vi "Functional data-Extract and save.vi"(7 "Simulate":bool, 8 "error in (no error)":errorcluster, 11 "Element received in the queue":T1={"Imaging Protocol"=enum."Live Imaging", "Number of Trials"=0, "Frame Size"=512, "# Averaged frames"=0, "Dwell time (us)"=0.0, "Index of Z-plane"=0, "Timelapse?"=FALSE, "Logging process is active"=FALSE, "Speed logging enabled"=FALSE, "tdms file ref"=refnum, "path"=path "", "Trial Number"=0, "Expected # points acquired"=FALSE, "Manually stopped"=FALSE, "Last trial"=FALSE, "Ch0 data"=[], "Ch1 data"=[], "Ref Data"=[], "Ref Frame Time"=[], "Image Time"=[], "Continuous Time"=[], "Ref X Length"=0, "Ref Y Length"=0, "# Ref Averaged frames"=0, "Ref Dwell time (us)"=0.0, "Points acquired"={"Ch0 last trial"=0, "Ch1 last trial"=0, "All trials"=0}, "HW Timings File"=refnum} {"Ref Dwell time (us)" format="%#.6g"; "Frame Size" items=["100X100"=100, "128X128"=128, "200X200"=200, "256X256"=256, "512X512"=512, "1024x1024"=1024, "2048x2048"=2048]; "Dwell time (us)" format="%#.6g"}) -> (0 "error out":errorcluster, 2 "Destination folder":path)   [LabVIEW 2020]
uses:
  Typedefs/Logging queue element.ctl
  Typedefs/Imaging Protocols enum.ctl
  Typedefs/Frame Size.ctl
  Typedefs/Acquired points count.ctl
  User Interface/Visualisation/Functional Imaging Viewer/SubVIs/Experiment header interface/Typedefs/Header file interface module functions enum.ctl
  User Interface/Visualisation/Functional Imaging Viewer/Typedefs/ROI Save interface cluster.ctl
panel:
  out "size(s) 2":i32[](array[numeric])
  out "ROI Data (header removed)":dbl[][](array[numeric])
  out "Functional imaging TDMS file path & name":path
  out "size(s)":i32[](array[numeric])
  out "No.of Cycles":i32
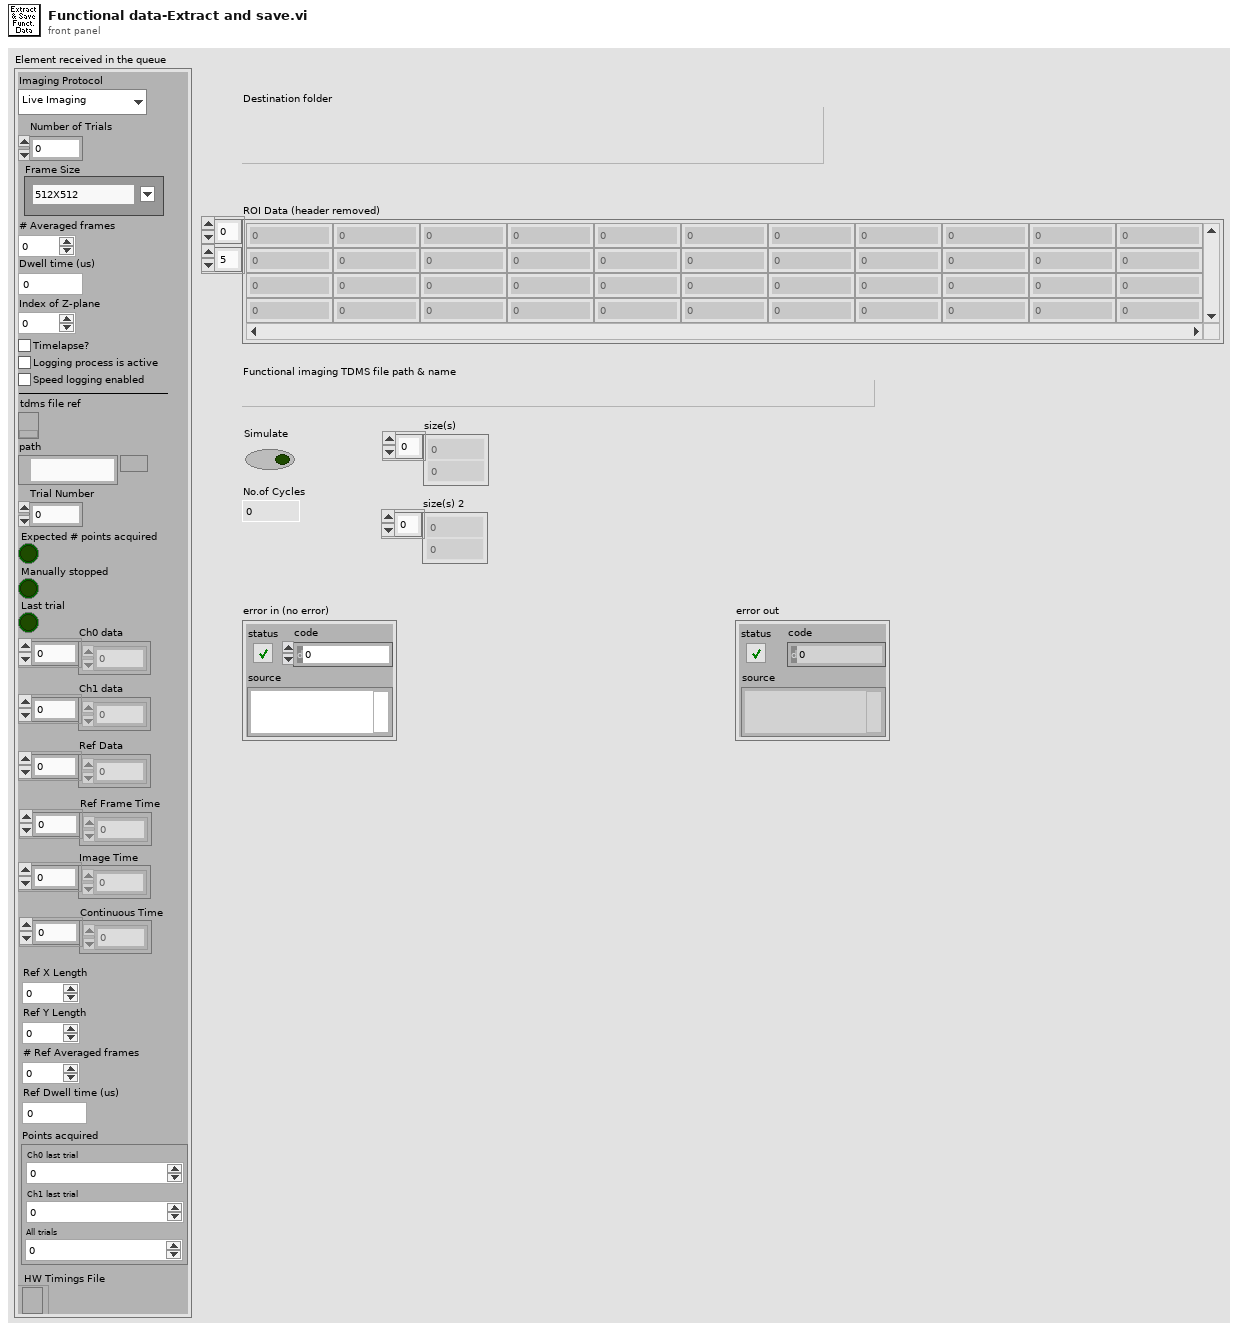
[diagram p1: front panel]
types:
  T1 = typedef "Logging queue element.ctl" = cluster{"Imaging Protocol":T2, "Number of Trials":u16, "Frame Size":T3, "# Averaged frames":u16, "Dwell time (us)":dbl, "Index of Z-plane":i32, "Timelapse?":bool, "Logging process is active":bool, "Speed logging enabled":bool, "tdms file ref":refnum<k34>, "path":path, "Trial Number":i32, "Expected # points acquired":bool, "Manually stopped":bool, "Last trial":bool, "Ch0 data":u32[], "Ch1 data":u32[], "Ref Data":u32[], "Ref Frame Time":u64[], "Image Time":u64[], "Continuous Time":u64[], "Ref X Length":u16, "Ref Y Length":u16, "# Ref Averaged frames":u16, "Ref Dwell time (us)":dbl, "Points acquired":T4, "HW Timings File":refnum<file>}
  T2 = typedef "Imaging Protocols enum.ctl" = enum16{"AOL Z-Stack", "Motor Z Stack", "Functional Acquisition", "Single Plane Acquisition", "Volume Acquisition", "Live Imaging", "Live Plane Imaging", "Live Volume Imaging"}
  T3 = typedef "Frame Size.ctl" = u16
  T4 = typedef "Acquired points count.ctl" = cluster{"Ch0 last trial":u64, "Ch1 last trial":u64, "All trials":u64}
  T5 = typedef "Header file interface module functions enum.ctl" = enum16{"Load experiment header file", "Save experiment header file", "Clear stored values", "Read stored values", "Update specific value in memory", "Update values in memory"}
  T6 = typedef "Header parameters cluster-ALL.ctl" = cluster{"LOGIN":T7, "GLOBAL PARAMETERS":T8, "IMAGING MODES":T10, "TIME SERIES":T11, "MOTOR Z-STACK ":T13, "AOL Z-STACK":T14, "FUNCTIONAL IMAGING":T15, "VOLUME IMAGING":T15, "MOVEMENT CORRECTION":T19, "CALIBRATION":T21, "STATISTICS":T22, "BIOLOGY INFORMATION":T23, "Calibration Data":T24}
  T7 = typedef "Header params -Login.ctl" = cluster{"User":string, "Profile":string, "Software Version":string, "Experiment Date Time":timestamp}
  T8 = typedef "Header params-Global Parameters.ctl" = cluster{"MicroscopeID":string, "Microscope Type":string, "Objective":string, "Field of View (um)":dbl, "Fill time (us)":dbl, "Experiment Type":T9, "Stimuli Trigger":bool, "Speed Logging":bool}
  T9 = typedef "Experiment Type.ctl" = enum16{"In vivo", "In vitro", "Testing", "Calibration", "Other"}
  T10 = typedef "Header params-Imaging Modes.ctl" = cluster{"Time Series":bool, "Motor Zstack":bool, "AOL Zstack":bool, "Functional Imaging":bool, "Volume Imaging":bool}
  T11 = typedef "Header params-Time Series.ctl" = cluster{"Basic Image meta data":T12, "AOL z":dbl}
  T12 = typedef "Header params-Basic image meta data.ctl" = cluster{"Wavelength (nm)":dbl, "# averaged frames":dbl, "laser power (%)":dbl, "Pockels":dbl, "pixel dwell time (us)":dbl, "pmt 1":dbl, "pmt 2":dbl, "back apperture":dbl, "zoom":dbl, "field of view":dbl, "Frame Size":T3, "AOL x centre":dbl, "AOL y centre":dbl, "Stage x position":dbl, "Stage y position":dbl, "Stage z position":dbl}
  T13 = typedef "Header params-Motor Z-stack.ctl" = cluster{"Hdr Basic Image meta data":T12, "Z Start":dbl, "Z Stop":dbl, "No of Planes":i32, "Laser Power (%) at Z Start":dbl, "Laser Power (%) at Z Stop":dbl}
  T14 = typedef "Header params-AOL Z-stack.ctl" = cluster{"Hdr Basic Image meta data":T12, "Z Start":dbl, "Z Stop":dbl, "No of Planes":i32, "Laser Power (%) at Z Start":dbl, "Laser Power (%) at Z Stop":dbl}
  T15 = typedef "Header params-Functional Imaging.ctl" = cluster{"Functional Mode":T16, "Variable Length":bool, "Variable Resolution":bool, "Pockels Modulation":bool, "Stimuli Trigger":bool, "Cool down enabled":bool, "AOL Mode":T17, "Plane Mode":T18, "Miniscan Dwell time per pixel (us)":dbl, "poi dwell time":dbl, "Number of trials":dbl, "Number of cycles":dbl, "Number of pois":dbl, "Number of miniscans":dbl, "Number of pixels in miniscan":dbl, "Rectangle ROI length":dbl, "Rectangle ROI height":dbl, "Frame rate (fps)":dbl, "Acquisition Length":dbl, "video length (sec)":dbl, "Stimuli delay (sec)":dbl, "Cool down time (sec)":dbl, "Basic Image meta data":T12, "Z Start (um)":dbl, "Z Stop (um)":dbl}
  T16 = typedef "Functional Mode.ctl" = enum16{"Point", "Line", "Patch", "Plane", "Volume"}
  T17 = typedef "AOL modes.ctl" = enum16{"Raster", "Structural", "Pointing", "Mini Scan", "Alignment"}
  T18 = typedef "Plane Mode.ctl" = u16
  T19 = typedef "Header params-Movement correction.ctl" = cluster{"Movement Correction":bool, "Axial Reference":bool, "Reference Source":T20, "Full Frame Size":dbl, "Reference Field of View":dbl, "Reference Zoom":dbl, "Reference dwell time (us)":dbl, "Reference X Pixels":dbl, "Reference Y Pixels":dbl, "Number of Z lines":dbl, "Size of Z pixels":dbl, "Axial Pixels":dbl, "Ignore Z lines":dbl, "Reference Scan Cycles":dbl, "Reference Threshold XY":dbl, "Reference Threshold Z":dbl, "Reference Average XY":dbl, "Reference Average Z":dbl, "Proportional Scale":dbl, "Integral Scale":dbl, "Proportional Scale Z":dbl, "Integral Scale Z":dbl, "Diff Threshold":dbl, "Diff Threshold Z":dbl, "Sliding Average":bool, "Reference count reset enabled":bool, "Scan Interval (ms)":dbl, "Ref Plot Refresh Rate (ms)":dbl}
  T20 = typedef "Reference source.ctl" = enum16{"Green channel", "Red channel"}
  T21 = typedef "Header params-Calibration Setup.ctl" = cluster{"Pockels Calibration File":path, "Calibration_ini file":path, "Setup_ini file":path}
  T22 = typedef "Header params-statistics.ctl" = cluster{"Z-stack duration (sec)":dbl, "Number of acquired data-points":dbl, "Acquisition time (ms)":dbl, "Number of acquired frames":dbl, "Intertrial times":dbl[]}
  T23 = typedef "Biology Information.ctl" = cluster{"Animal Code or Name":string, "Animal DoB":string, "Animal Age":string, "Animal Sex":string, "Animal Weight":string, "Date of Injection":string, "Date of Implant":string, "Site of Injection":string, "Animal Ear Notch":string, "AAV constructs":string, "Genetic background":string, "Optical reporter":string, "Region of brain imaged":string, "Other \ncomments":string}
  T24 = typedef "Header params-calibration data.ctl" = cluster{"Objective Name":string, "Calibration Wavelength":dbl, "Sum X":dbl, "Sum Y":dbl, "Diff X":dbl, "Diff Y":dbl, "Distortion Correction":dbl, " Z norm to um Scaling":dbl, " X norm to um Scaling":dbl}
  T25 = typedef "ROI Save interface cluster.ctl" = cluster{"Trial Number (unity-based)":i32, "ROI Index (zero-based)":i32, "ROI ID":i32, "ROI Time (ns)":i32, "# of Pixels in ROI":i32, "Channel No. (unity based)":i32}
  T26 = typedef "Fixed strings.ctl" = cluster{"ROI file name":string, "Normalised ROI file name":string, "Zplane Pockels values file name":string, "Functional data folder name":string, "Experiment Header file name":string, "Z-stack images folder name":string, "Groups setup rel. path":string, "Groups text file rel. path":string, "TDMS files folder name (F.img)":string, "TDMS files folder name (V.acq)":string, "TDMS files folder name (Pl.acq)":string, "Cycle rel times sequence file":string, "Dynamically called VIs folder name":string, "Time Series folder base name":string}
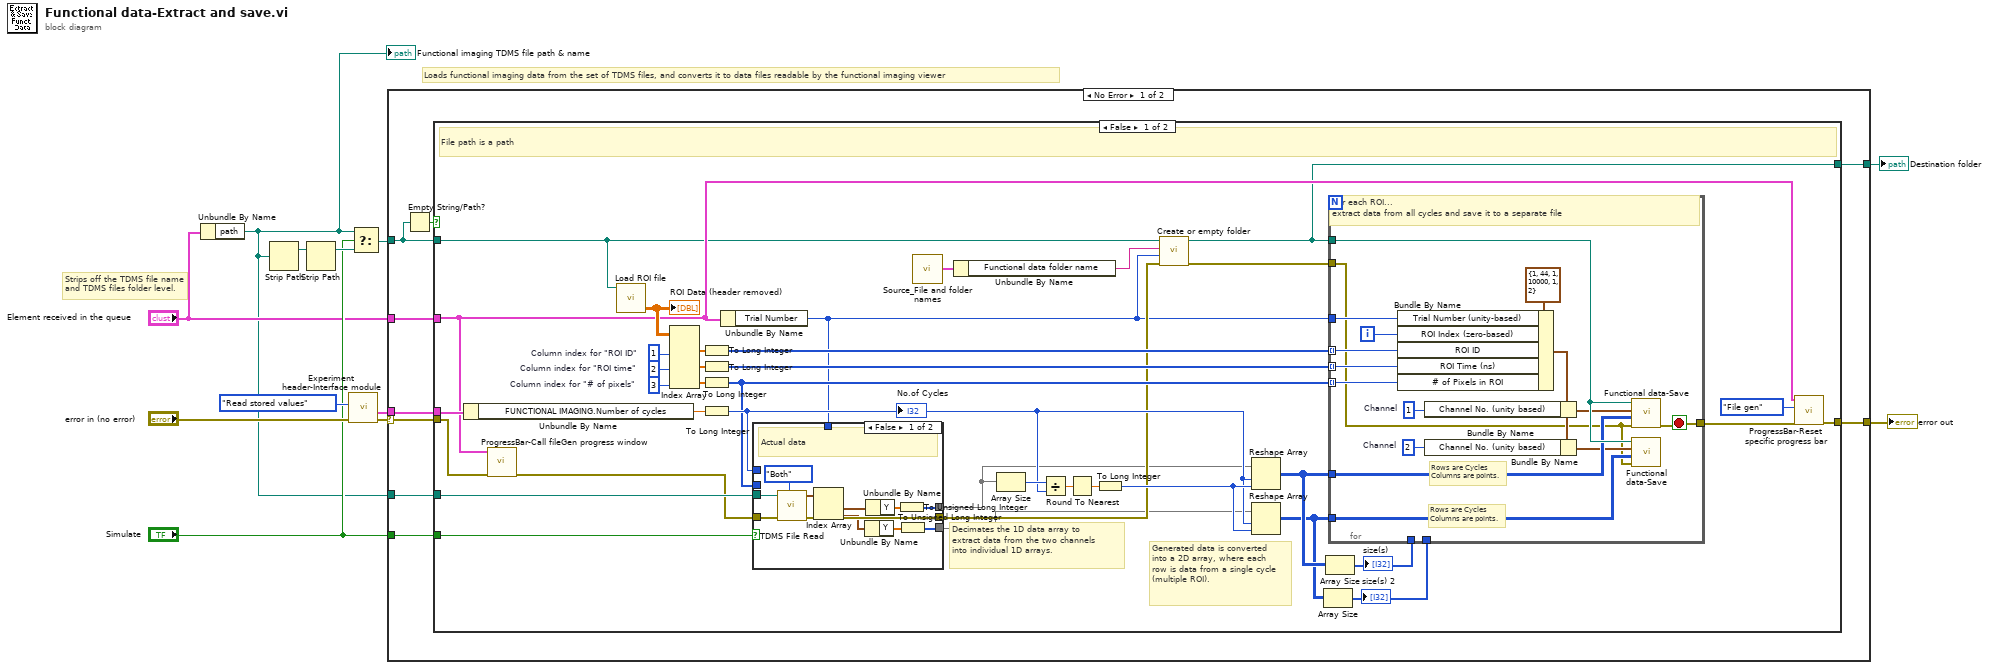
[diagram p0: block diagram]
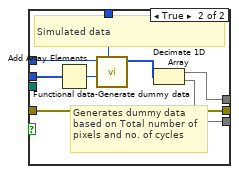
[diagram p2: hidden frame]
diagram:
  # "Strips off the TDMS file name and TDMS files folder level."
  # "Loads functional imaging data from the set of TDMS files, and converts it to data files readable by the functional imaging viewer"
  n1 = Unbundle By Name("Element received in the queue") -> ("path"=w2:path)
  "Functional imaging TDMS file path & name" <- w2
  n2 = Strip Path(path=w2) -> (stripped path=w7:path)  [unwired: 1 out]
  n3 = Strip Path(path=w7) -> (stripped path=w6:path)  [unwired: 1 out]
  n4 = call "Experiment header-Interface module.vi"("error in (no error)"="error in (no error)", "Function"=Header_file_interface_module_functions_enum."Read stored values") -> ("error out"=w9:errorcluster, "All header parameters out"=w8:T6)  [unwired: 8 in]
  n5 = Select(t=w2, s="Simulate", f=w6) -> (s? t:f=w5:path)
  n6 = case shown="No Error" w9 {
    selector: w9 -> [w18 w96]
    tunnel: [w17 w96] -> w12
    tunnel: "Element received in the queue" -> [w14 _]
    tunnel: w5 -> [w20 _]
    tunnel: "Simulate" -> [w21 _]
    tunnel: w8 -> [w16 _]
    tunnel: w2 -> [w15 _]
    tunnel: [w13 _] -> w1
    frame No Error {
      n7 = Empty String/Path?(string/path=w20) -> (empty?=w19:bool)
      n8 = case shown="False" w19 {
        tunnel: w21 -> [w52 _]
        tunnel: w14 -> [w34 _]
        tunnel: w20 -> [w33 _]
        tunnel: w18 -> [w39 w95]
        tunnel: [w36 w95] -> w17
        tunnel: w16 -> [w41 _]
        tunnel: w15 -> [w40 _]
        tunnel: [w24 _] -> w13
        frame False {
          w49 = 2  # Column index for "ROI time"
          w50 = 3  # Column index for "# of pixels"
          w59 = 1  # Column index for "ROI ID"
          # "Decimates the 1D data array to extract data from the two channels into individual 1D arrays."
          # "Generated data is converted into a 2D array, where each row is data from a single cycle (multiple ROI)."
          # "File path is a path"
          n9 = Unbundle By Name(w41) -> ("FUNCTIONAL IMAGING.Number of cycles"=w54:dbl)
          n10 = call "ProgressBar-Call fileGen progress window.vi"("error in (no error)"=w39, "Z-stack queue cluster"=w34) -> ("error out"=w38:errorcluster)  [unwired: 9 in]
          n11 = call "Load ROI file.vi"("Experiment data folder path"=w33) -> ("ROI Data (header removed)"=w53:dbl[][])  [unwired: 7 in, 3 out]
          "ROI Data (header removed)" <- w53
          n12 = Index Array(array=w53, index (col) #1=w59, index (col) #2=w49, index (col) #3=w50) -> (element #1=w48:dbl[], element #2=w47:dbl[], element #3=w43:dbl[])  [unwired: 3 in]
          n13 = To Long Integer(number=w48) -> (32bit integer=w46:i32[])
          n14 = To Long Integer(number=w47) -> (32bit integer=w45:i32[])
          n15 = To Long Integer(number=w43) -> (32bit integer=w44:i32[])
          n16 = To Long Integer(number=w54) -> (32bit integer=w51:i32)
          "No.of Cycles" <- w51
          n17 = Unbundle By Name(w34) -> ("Trial Number"=w30:i32)
          n18 = case shown="False" w52 {
            tunnel: [w67 w72] -> w22
            tunnel: w51 -> [_ w76]
            tunnel: w44 -> [_ w78]
            tunnel: w30 -> [_ w75]
            tunnel: w40 -> [w66 _]
            tunnel: w38 -> [w65 w74]
            tunnel: [w64 w74] -> w31
            tunnel: [w62 w71] -> w23
            frame False {
              # "Actual data"
              n19 = call "TDMS File Read.vi"("Error In"=w65, "Channel to load"=enum16{"Red", "Green", "Both"}."Both", "File Path"=w66) -> ("Error Out"=w64:errorcluster, "Data"=w70:waveform(dbl)[])  [unwired: 4 in, 3 out]
              n20 = Index Array(array=w70) -> (element #1=w69:waveform(dbl), element #2=w63:waveform(dbl))  [unwired: 2 in]
              n21 = Unbundle By Name(w63) -> ("Y"=w61:dbl[])
              n22 = Unbundle By Name(w69) -> ("Y"=w68:dbl[])
              n23 = To Unsigned Long Integer(number=w68) -> (unsigned 32bit integer=w67:u32[])
              n24 = To Unsigned Long Integer(number=w61) -> (unsigned 32bit integer=w62:u32[])
            }
            frame True {
              # "Generates dummy data based on Total number of pixels and no. of cycles"
              # "Simulated data"
              n25 = Add Array Elements(numeric array=w78) -> (sum=w77:i32)
              n26 = call "Functional data-Generate dummy data.vi"("Trial number (unity-based)"=w75, "total no. of points in each cycle"=w77, "no. of  cycles"=w76) -> ("Single trial data (inc. POIs and miniscans, multiple cycles)"=w73:u32[])  [unwired: 8 in]
              n27 = Decimate 1D Array(w73) -> (w72:u32[], w71:u32[])
            }
          }
          n28 = call "Source_File and folder names.vi"() -> ("Fixed strings"=w29:T26)  [unwired: 1 in]
          n29 = Unbundle By Name(w29) -> ("Functional data folder name"=w28:string)
          n30 = Array Size(array=w22) -> (size(s)=w58:i32)
          n31 = Divide(x=w58, y=w51) -> (x/y=w57:dbl)
          n32 = Round To Nearest(number=w57) -> (nearest integer value=w56:dbl)
          n33 = To Long Integer(number=w56) -> (32bit integer=w55:i32)
          n34 = call "Create or empty folder.vi"("error in (no error)"=w31, "Trial Number"=w30, "name of folder to create or empty"=w28, "Experiment folder path"=w33) -> ("error out"=w32:errorcluster, "appended path"=w24:path)  [unwired: 6 in]
          n35 = Reshape Array "Reshape Array"(w22, w51, w55) -> (w42:u32[][])
          n36 = Reshape Array(w23, w51, w55) -> (w26:u32[][])
          n37 = Array Size(array=w26) -> (size(s)=w25:i32[])
          "size(s) 2" <- w25
          n38 = Array Size(array=w42) -> (size(s)=w27:i32[])
          "size(s)" <- w27
          n39 = for {
            tunnel: w42 -> [w88]
            tunnel: w46 -> [w91] mode=indexing
            tunnel: w44 -> [w89] mode=indexing
            tunnel: w24 -> [w92]
            tunnel: w30 -> [w81]
            tunnel: w26 -> [w86]
            tunnel: w45 -> [w90] mode=indexing
            tunnel: [w79] -> w35
            tunnel: w32 -> [w80]
            tunnel: w27 -> [_]
            tunnel: w25 -> [_]
            i -> [w82]
            stop <- w79 stop-if-true
            w93 = 2  # Channel
            w84 = 1  # Channel
            # "Rows are Cycles\nColumns are points."
            # "Rows are Cycles\nColumns are points."
            # "For each ROI... \nextract data from all cycles and save it to a separate file"
            n40 = Bundle By Name(cluster=T25 {"Trial Number (unity-based)"=1, "ROI Index (zero-based)"=44, "ROI ID"=1, "ROI Time (ns)"=10000, "# of Pixels in ROI"=1, "Channel No. (unity based)"=2} ("ROI Save interface cluster"), "Trial Number (unity-based)"=w81, "ROI Index (zero-based)"=w82, "ROI ID"=w91, "ROI Time (ns)"=w90, "# of Pixels in ROI"=w89) -> (w83:T25)
            n41 = Bundle By Name(cluster=w83, "Channel No. (unity based)"=w84) -> (w85:T25)
            n42 = Bundle By Name(cluster=w83, "Channel No. (unity based)"=w93) -> (w87:T25)
            n43 = call "Functional data-Save.vi"("error in"=w80, "Reshaped Array"=w88, "ROI Save interface cluster"=w85, "Data folder path"=w92) -> ("error out"=w79:errorcluster)  [unwired: 7 in]
            n44 = call "Functional data-Save.vi"("error in"=w80, "Reshaped Array"=w86, "ROI Save interface cluster"=w87, "Data folder path"=w92) -> ()  [unwired: 7 in, 1 out]
          }
          n45 = call "ProgressBar-Reset specific progress bar.vi"("Error in"=w35, "Sender"=enum16{"Acquisition", "Logging", "File gen"}."File gen", "Z-stack queue cluster"=w34) -> ("error out"=w36:errorcluster)  [unwired: 8 in]
        }
        frame True {
          # "File path is empty or not a path"
        }
      }
    }
    frame Error {
    }
  }
  "error out" <- w12
  "Destination folder" <- w1
